vi "CreateNotifier.vi"(8 "entrée d'erreur (pas d'erreur)":errorcluster) -> (0 "sortie d'erreur":errorcluster, 3 "Notifiers":T1)   [LabVIEW 2017, in "Notifier.lvlib"]
doc: "Ce VI crée tous les notifier liés à chaque appareils du centre d'usinage.\nPour l'ajout ou le retrait d'un appareil, il faut modifier ce VI.\nOn retrouve en entrée, le cluster d'erreur ; en sortie, un cluster regroupant les notifiers de chaque appareils nommer par la CTL \"notifier.ctl\", le cluster d'erreur de sortie."
uses:
  Notifier.lvlib
  Notifier.ctl
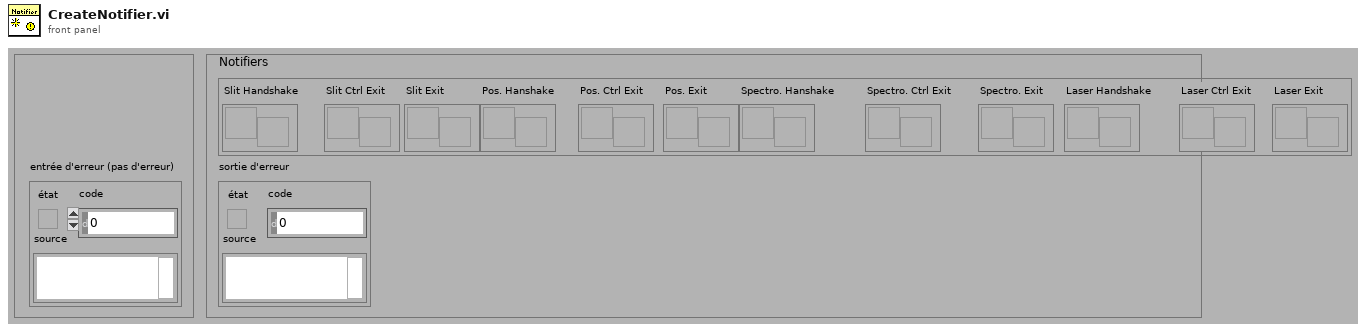
[diagram p1: front panel]
types:
  T1 = typedef "Notifier.lvlib/Notifier.ctl" = cluster{"Slit Handshake":refnum<notifier>, "Slit Ctrl Exit":refnum<notifier>, "Slit Exit":refnum<notifier>, "Pos. Hanshake":refnum<notifier>, "Pos. Ctrl Exit":refnum<notifier>, "Pos. Exit":refnum<notifier>, "Spectro. Hanshake":refnum<notifier>, "Spectro. Ctrl Exit":refnum<notifier>, "Spectro. Exit":refnum<notifier>, "Laser Handshake":refnum<notifier>, "Laser Ctrl Exit":refnum<notifier>, "Laser Exit":refnum<notifier>}
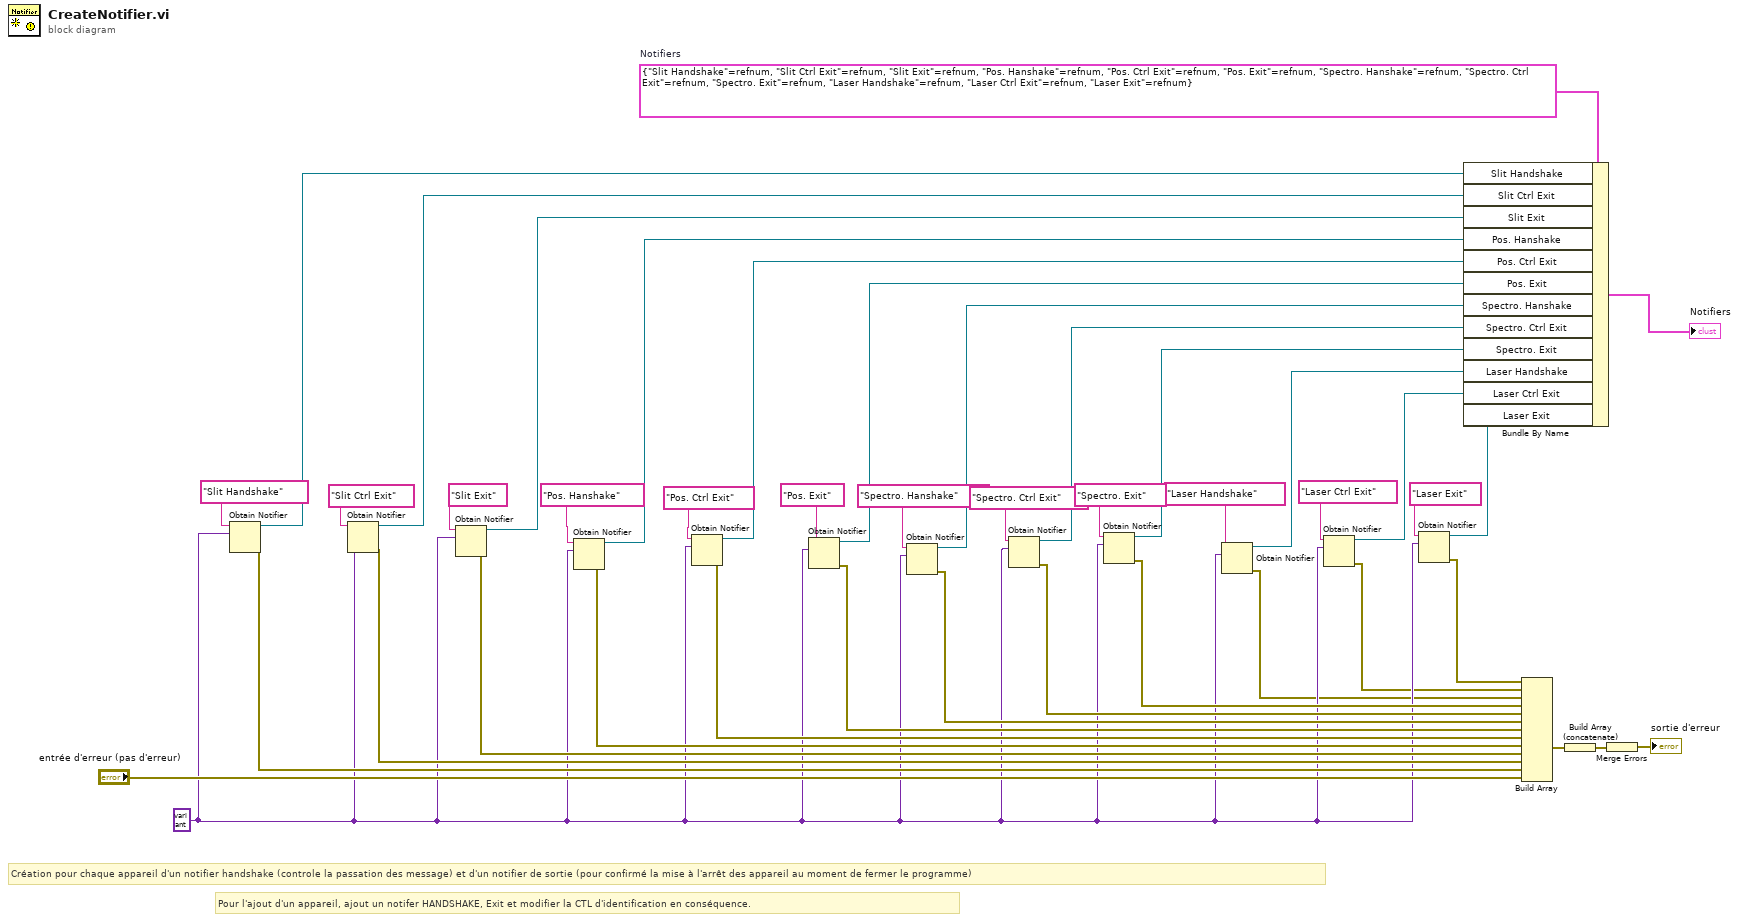
[diagram p0: block diagram]
diagram:
  w38 = T1 {"Slit Handshake"=refnum, "Slit Ctrl Exit"=refnum, "Slit Exit"=refnum, "Pos. Hanshake"=refnum, "Pos. Ctrl Exit"=refnum, "Pos. Exit"=refnum, "Spectro. Hanshake"=refnum, "Spectro. Ctrl Exit"=refnum, "Spectro. Exit"=refnum, "Laser Handshake"=refnum, "Laser Ctrl Exit"=refnum, "Laser Exit"=refnum}  # Notifiers
  w8 = variant ("variant")
  # "Pour l'ajout d'un appareil, ajout un notifer HANDSHAKE, Exit et modifier la CTL d'identification en conséquence."
  # "Création pour chaque appareil d'un notifier handshake (controle la passation des message) et d'un notifier de sortie (pour confirmé la mise à l'arrêt des appareil au moment de fermer le programme)"
  n1 = Obtain Notifier(name (unnamed)="Slit Handshake" ("nom (aucun)"), notification data type=w8) -> (notifier out=w43:refnum<notifier>, error out=w41:errorcluster)  [unwired: 2 in, 1 out]
  n2 = Obtain Notifier(name (unnamed)="Slit Ctrl Exit" ("nom (aucun)"), notification data type=w8) -> (notifier out=w34:refnum<notifier>, error out=w36:errorcluster)  [unwired: 2 in, 1 out]
  n3 = Obtain Notifier(name (unnamed)="Slit Exit" ("nom (aucun)"), notification data type=w8) -> (notifier out=w33:refnum<notifier>, error out=w35:errorcluster)  [unwired: 2 in, 1 out]
  n4 = Obtain Notifier(name (unnamed)="Pos. Hanshake" ("nom (aucun)"), notification data type=w8) -> (notifier out=w32:refnum<notifier>, error out=w30:errorcluster)  [unwired: 2 in, 1 out]
  n5 = Obtain Notifier(name (unnamed)="Pos. Ctrl Exit" ("nom (aucun)"), notification data type=w8) -> (notifier out=w31:refnum<notifier>, error out=w29:errorcluster)  [unwired: 2 in, 1 out]
  n6 = Obtain Notifier(name (unnamed)="Pos. Exit" ("nom (aucun)"), notification data type=w8) -> (notifier out=w28:refnum<notifier>, error out=w24:errorcluster)  [unwired: 2 in, 1 out]
  n7 = Obtain Notifier(name (unnamed)="Spectro. Hanshake" ("nom (aucun)"), notification data type=w8) -> (notifier out=w27:refnum<notifier>, error out=w23:errorcluster)  [unwired: 2 in, 1 out]
  n8 = Obtain Notifier(name (unnamed)="Spectro. Ctrl Exit" ("nom (aucun)"), notification data type=w8) -> (notifier out=w26:refnum<notifier>, error out=w22:errorcluster)  [unwired: 2 in, 1 out]
  n9 = Obtain Notifier(name (unnamed)="Spectro. Exit" ("nom (aucun)"), notification data type=w8) -> (notifier out=w25:refnum<notifier>, error out=w21:errorcluster)  [unwired: 2 in, 1 out]
  n10 = Obtain Notifier(name (unnamed)="Laser Handshake" ("nom (aucun)"), notification data type=w8) -> (notifier out=w6:refnum<notifier>, error out=w3:errorcluster)  [unwired: 2 in, 1 out]
  n11 = Obtain Notifier(name (unnamed)="Laser Ctrl Exit" ("nom (aucun)"), notification data type=w8) -> (notifier out=w5:refnum<notifier>, error out=w2:errorcluster)  [unwired: 2 in, 1 out]
  n12 = Obtain Notifier(name (unnamed)="Laser Exit" ("nom (aucun)"), notification data type=w8) -> (notifier out=w4:refnum<notifier>, error out=w1:errorcluster)  [unwired: 2 in, 1 out]
  n13 = Bundle By Name(cluster=w38, "Slit Handshake"=w43, "Slit Ctrl Exit"=w34, "Slit Exit"=w33, "Pos. Hanshake"=w32, "Pos. Ctrl Exit"=w31, "Pos. Exit"=w28, "Spectro. Hanshake"=w27, "Spectro. Ctrl Exit"=w26, "Spectro. Exit"=w25, "Laser Handshake"=w6, "Laser Ctrl Exit"=w5, "Laser Exit"=w4) -> (→"Notifiers":T1)
  n14 = Build Array(w1, w2, w3, w21, w22, w23, w24, w29, w30, w35, w36, w41, "entrée d'erreur (pas d'erreur)") -> (w42:errorcluster[])
  n15 = Build Array (concatenate)(w42) -> (w37:errorcluster[])
  n16 = Merge Errors(w37) -> (→"sortie d'erreur":errorcluster)
